vi "AI RTM Enable Disable.vi"(8 "error in (no error)":errorcluster, 11 "Node Ref":T1 format="%.0x") -> (0 "error out":errorcluster)   [LabVIEW 2013]
uses:
  <vilib>/K2Labs/HiLab API/Custom Device API/Controls/Custom Device Item Reference.ctl
  <vilib>/K2Labs/HiLab API/Custom Device API/Configuration/Item Properties/Get Item Property/Get Item Property.xnode
  <vilib>/K2Labs/HiLab API/Custom Device API/Configuration/Item Properties/Set Item Property/Set Item Property.xnode
  <vilib>/K2Labs/HiLab API/Custom Device API/Custom Device API Library.lvlib
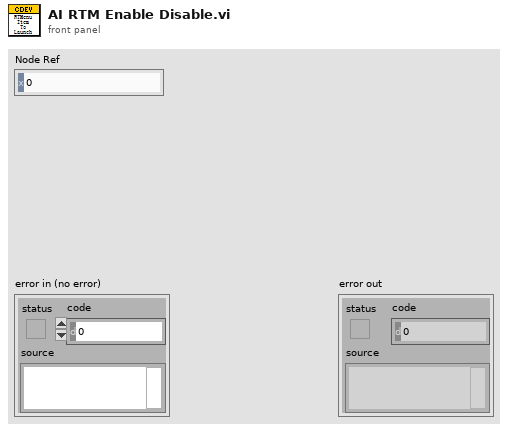
[diagram p1: front panel]
types:
  T1 = typedef "Custom Device API Library.lvlib/Custom Device Item Reference.ctl" = u64
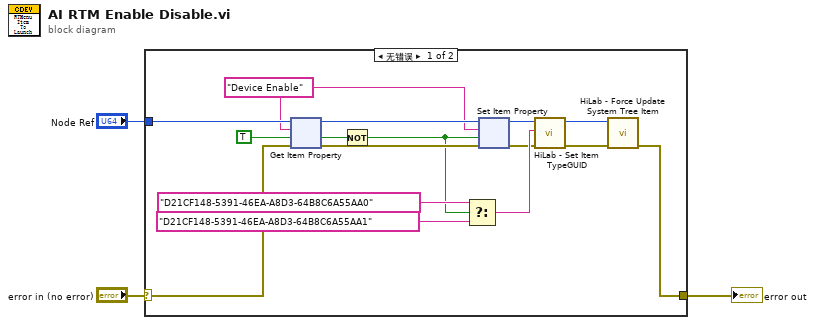
[diagram p0: block diagram]
diagram:
  n1 = case shown="无错误" "error in (no error)" {
    selector: "error in (no error)" -> [w12 w79]
    tunnel: [w17 w79] -> w2
    tunnel: "Node Ref" -> [w13 _]
    frame No Error {
      w10 = "Device Enable" ("Property Name")
      n2 = xnode "Get Item Property"("Item Ref in"=w13, "Property Name"=w10, "Default Value"=TRUE, "error in (no error)"=w12) -> ("Item Ref out"=w11:T1, "Value"=w5:bool, "error out"=w8:errorcluster)  [unwired: 1 out]
      n3 = Not(x=w5) -> (.not. x?=w4:bool)
      n4 = Select(t="D21CF148-5391-46EA-A8D3-64B8C6A55AA0" ("TypeGUID"), s=w4, f="D21CF148-5391-46EA-A8D3-64B8C6A55AA1" ("TypeGUID")) -> (s? t:f=w14:string)
      n5 = xnode "Set Item Property"("Item Ref in"=w11, "error in (no error)"=w8, "Property Name"=w10, "Value"=w4) -> ("Item Ref out"=w6:T1, "error out"=w7:errorcluster)  [unwired: 1 out]
      n6 = call <vilib>:"HiLab - Set Item TypeGUID.vi"("error in (no error)"=w7, "TypeGUID"=w14, "Item Ref in"=w6) -> ("error out"=w18:errorcluster, "Item Ref out"=w19:T1)  [unwired: 7 in]
      n7 = call <vilib>:"HiLab - Force Update System Tree Item.vi"("error in (no error)"=w18, "Item Ref in"=w19) -> ("error out"=w17:errorcluster)  [unwired: 8 in, 1 out]
    }
    frame Error {
    }
  }
  "error out" <- w2
